vi "LVFunction_Imop_GetExePathToConvertionTools.vi"(11 "error in (no error)":errorcluster) -> (4 "ExePath":path)   [LabVIEW 2020]
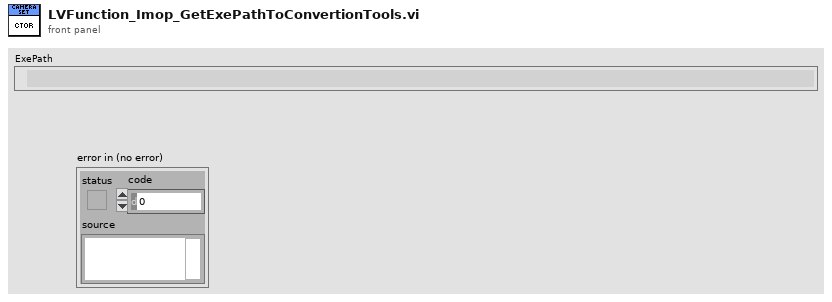
[diagram p1: front panel]
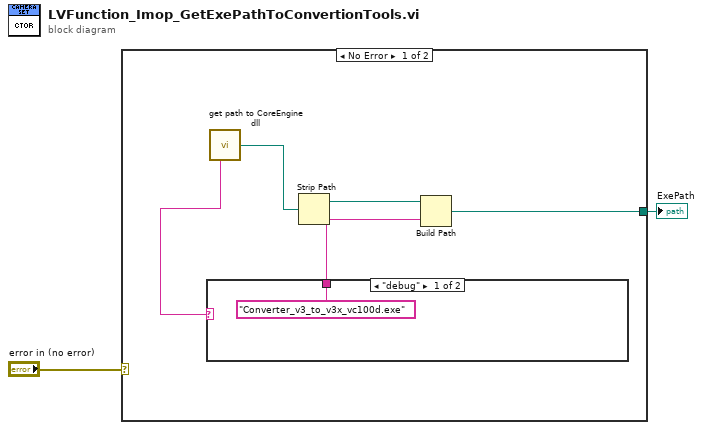
[diagram p0: block diagram]
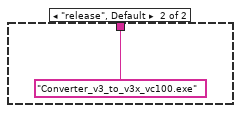
[diagram p2: hidden frame]
diagram:
  n1 = case shown="No Error" "error in (no error)" {
    tunnel: [w5 _] -> w1
    frame No Error {
      n2 = call "get path to CoreEngine dll.vi"() -> ("path to c_interface_vc100.dll"=w7:path, "Release/Debug"=w3:string)  [unwired: 12 in, 2 out]
      n3 = case shown="\"debug\"" w3 {
        tunnel: ["Converter_v3_to_v3x_vc100d.exe" ("name or relative path") "Converter_v3_to_v3x_vc100.exe" ("name or relative path")] -> w4
        frame "debug" {
        }
        frame "release", Default {
        }
      }
      n4 = Strip Path(path=w7) -> (stripped path=w6:path)  [unwired: 1 out]
      n5 = Build Path(base path=w6, name or relative path=w4) -> (appended path=w5:path)
    }
    frame Error {
    }
  }
  "ExePath" <- w1
